vi "SetSystemTime.vi"(0 "Time and Date":T1, 7 "Is UTC?":bool=TRUE caption="Is UTC? (T)", 11 "Error in":errorcluster caption="Error in (no error)") -> (15 "Error out":errorcluster)   [LabVIEW 2017, in "GPTiming.lvlib"]
doc: "Sets a new system <B>Time and Date</B>.\n\nThis VI sets the time and date directly in Windows (<B>thus this VI is Windows only</B>). Since LabVIEW does not register if the time zone has changed at runtime, this VI can be necessary in applications where the time, date and/or timezone is changed manually or programmatically at runtime.\n\nIf <B>Is UTC?</B> is True (default) the time is assumed to be a UTC time. If <B>Is UTC?</B> is False the time is assumed to be in the local system time zone and DST observation.\n\n<B>Setting the system time and date requires elevated privileges in Windows, usually best achieved by running LabVIEW as administrator when using this VI.</B>\n\nThis VI runs only if there is no error on <B>Error in</B>.\n\nSteen Schmidt\nGPower\n4/2 2017"
uses:
  GPTiming.lvlib
  kernel32.dll
  Error/GPError.lvlib
  Date.ctl
  Time.ctl
  TimeAndDate.ctl
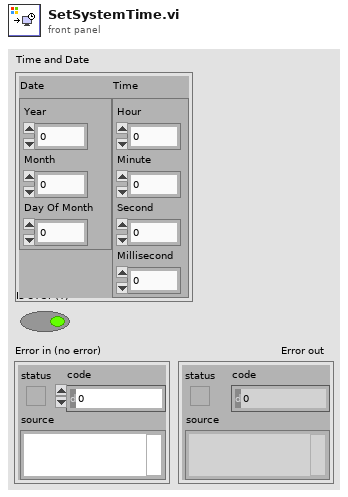
[diagram p1: front panel]
types:
  T1 = typedef "GPTiming.lvlib/TimeAndDate.ctl" = cluster{"Date":T2, "Time":T3}
  T2 = typedef "GPTiming.lvlib/Date.ctl" = cluster{"Year":u16, "Month":u16, "Day Of Month":u16}
  T3 = typedef "GPTiming.lvlib/Time.ctl" = cluster{"Hour":u16, "Minute":u16, "Second":u16, "Millisecond":u16}
  T4 = cluster{"Year":u16, "Month":u16, "Day of Week":u16, "Day of Month":u16, "Hour":u16, "Minute":u16, "Second":u16, "Millisecond":u16}
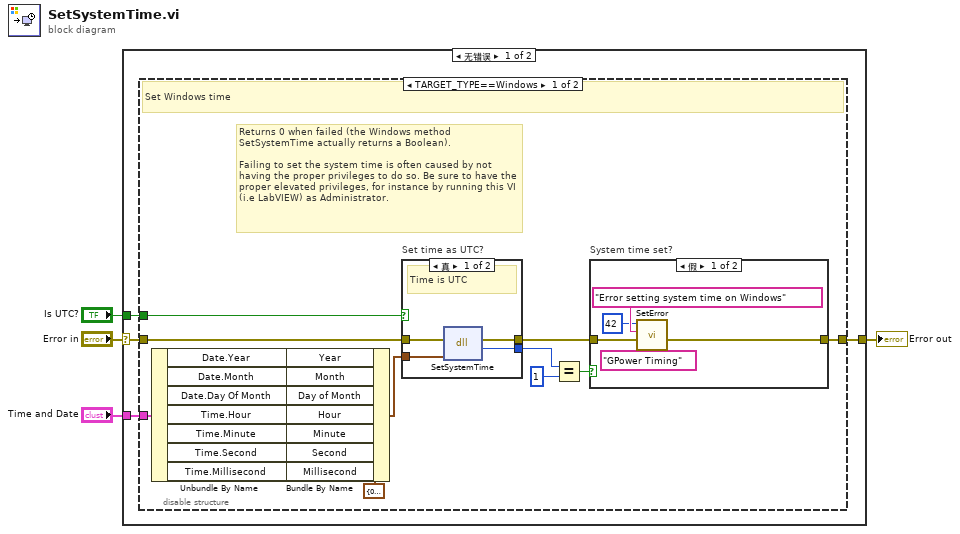
[diagram p0: block diagram]
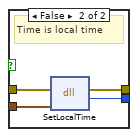
[diagram p2: hidden frame]
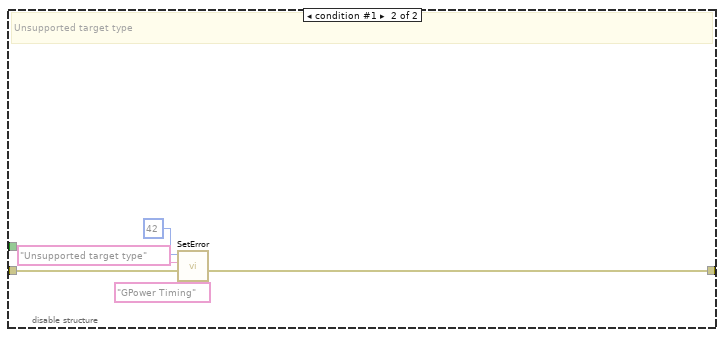
[diagram p4: hidden frame]
diagram:
  n1 = case shown="无错误" "Error in" {
    selector: "Error in" -> [w8 w45]
    tunnel: [w7 w45] -> w1
    tunnel: "Is UTC?" -> [w6 _]
    tunnel: "Time and Date" -> [w5 _]
    frame No Error {
      n2 = disable-structure shown="TARGET_TYPE==Windows" {
        disable-tunnel: w8 -> [w12 w42]
        disable-tunnel: [w11 w40] -> w7
        disable-tunnel: w6 -> [w10 _]
        disable-tunnel: w5 -> [w9 _]
        frame condition #0 (active) {
          # "Returns 0 when failed (the Windows method SetSystemTime actually returns a Boolean).\n\nFailing to set the system time is often caused by not having the proper privileges to do so. Be sure to have the proper elevated privileges, for instance by running this VI (i.e LabVIEW) as Administrator."
          # "Set Windows time"
          n3 = Unbundle By Name(w9) -> ("Date.Year"=w19:u16, "Date.Month"=w20:u16, "Date.Day Of Month"=w21:u16, "Time.Hour"=w22:u16, "Time.Minute"=w23:u16, "Time.Second"=w24:u16, "Time.Millisecond"=w25:u16)
          n4 = Bundle By Name(cluster=T4 {"Year"=0, "Month"=0, "Day of Week"=0, "Day of Month"=0, "Hour"=0, "Minute"=0, "Second"=0, "Millisecond"=0} ("System Time"), "Year"=w19, "Month"=w20, "Day of Month"=w21, "Hour"=w22, "Minute"=w23, "Second"=w24, "Millisecond"=w25) -> (w14:T4)
          n5 = case "Set time as UTC?" shown="真" w10 {
            tunnel: w14 -> [w29 w33]
            tunnel: [w28 w32] -> w15
            tunnel: w12 -> [w27 w31]
            tunnel: [w26 w30] -> w18
            frame True {
              # "Time is UTC"
              n6 = dll-call lib="kernel32.dll" fn="SetSystemTime"(error in=w27, "Time"=w29) -> (error out=w26:errorcluster, "return type"=w28:i8)  [unwired: 3 in, 1 out]
            }
            frame False {
              # "Time is local time"
              n7 = dll-call lib="kernel32.dll" fn="SetLocalTime"(error in=w31, "Time"=w33) -> (error out=w30:errorcluster, "return type"=w32:i8)  [unwired: 3 in, 1 out]
            }
          }
          n8 = Equal?(x=w15, y=i8 1) -> (x = y?=w17:bool)
          n9 = case "System time set?" shown="假" w17 {
            tunnel: w18 -> [w36 w39]
            tunnel: [w34 w39] -> w11
            frame False {
              n10 = call "SetError.vi"("Error label"="GPower Timing", "Error in"=w36, "Error description"="Error setting system time on Windows", "Error code"=42) -> ("Error out"=w34:errorcluster)  [unwired: 7 in]
            }
            frame True {
            }
          }
        }
        frame condition #1 {
          # "Unsupported target type"
          n11 = call "SetError.vi"("Error label"="GPower Timing", "Error in"=w42, "Error description"="Unsupported target type", "Error code"=42) -> ("Error out"=w40:errorcluster)  [unwired: 7 in]
        }
      }
    }
    frame Error {
    }
  }
  "Error out" <- w1
